vi "(nist) Post Joint Values.vi"(11 "Reply":string) -> ()   [LabVIEW 2013]
uses:
  (nist) Arm Globals.vi
panel:
  out "R":u32
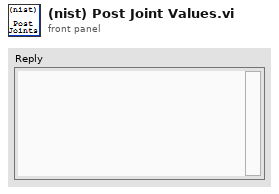
[diagram p1: front panel]
types:
  T1 = cluster{"Joint Names":string[], "Position":dbl[], "Velocity":dbl[], "Effort":dbl[]}
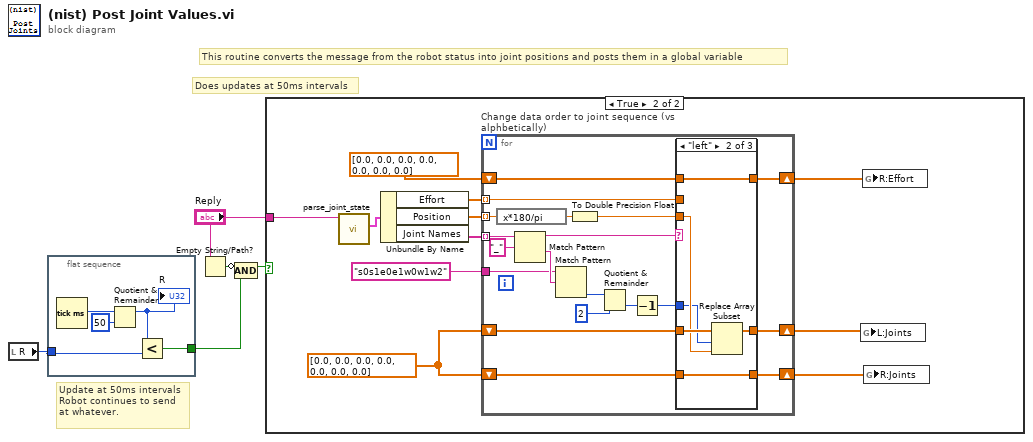
[diagram p0: block diagram]
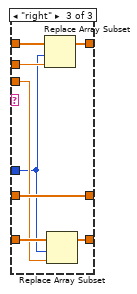
[diagram p4: hidden frame]
diagram:
  # "Update at 50ms intervals\nRobot continues to send\nat whatever."
  # "Does updates at 50ms intervals"
  # "This routine converts the message from the robot status into joint positions and posts them in a global variable"
  n1 = local read "R"() -> (w1:u32)
  n2 = flat-sequence {
    tunnel: [w7] -> w2
    tunnel: w1 -> [w6]
    frame #0 {
      n3 = Tick Count (ms)() -> (millisecond timer value=w10:u32)
      n4 = Quotient & Remainder(x=w10, y=u32 50) -> (x-y*floor(x/y)=w8:u32)  [unwired: 1 out]
      "R" <- w8
      n5 = Less?(x=w8, y=w6) -> (x < y?=w7:bool)
    }
  }
  n6 = Empty String/Path?(string/path="Reply") -> (empty?=w5:bool)
  n7 = Compound Arithmetic op=AND(invert w5, w2) -> (w3:bool)
  n8 = case shown="True" w3 {
    tunnel: "Reply" -> [_ w16]
    frame False {
    }
    frame True {
      w21 = dbl[] [0.0, 0.0, 0.0, 0.0, 0.0, 0.0, 0.0]
      n9 = call "parse_joint_state.vi"("msg in"=w16) -> ("ROS Joint States"=w19:T1)  [unwired: 3 in, 3 out]
      n10 = Unbundle By Name(w19) -> ("Effort"=w13:dbl[], "Position"=w18:dbl[], "Joint Names"=w17:string[])
      n11 = for "Change data order to joint sequence (vs alphbetically)" {
        shift-right: [w40] -> w14
        shift-left: w21 -> [w39]
        shift-right: [w37] -> w15
        shift-left: w21 -> [w38]
        tunnel: w17 -> [w33] mode=indexing
        tunnel: w18 -> [w36] mode=indexing
        tunnel: "s0s1e0e1w0w1w2" -> [w26]
        tunnel: w13 -> [w24] mode=indexing
        shift-right: [w23] -> w11
        shift-left: dbl[] [0.0, 0.0, 0.0, 0.0, 0.0, 0.0, 0.0] -> [w22]
        n12 = expression code="x*180/pi"(w36) -> (w35:dbl)
        n13 = Match Pattern(string=w33, regular expression="_") -> (before substring=w27:string, after substring=w31:string)  [unwired: 1 in, 2 out]
        n14 = Match Pattern(string=w26, regular expression=w31) -> (offset past match=w30:i32)  [unwired: 1 in, 3 out]
        n15 = To Double Precision Float(number=w35) -> (double precision float=w34:dbl)
        n16 = Quotient & Remainder(x=w30, y=2) -> (floor(x/y)=w28:i32)  [unwired: 1 out]
        n17 = Decrement(x=w28) -> (x-1=w25:i32)
        n18 = case shown="\"left\"" w27 {
          tunnel: [w43 w47 w57] -> w40
          tunnel: w39 -> [w43 w48 w57]
          tunnel: w34 -> [_ w46 w54]
          tunnel: w38 -> [w42 w49 w55]
          tunnel: [w42 w49 w56] -> w37
          tunnel: w25 -> [_ w45 w52]
          tunnel: w24 -> [_ _ w53]
          tunnel: [w41 w44 w51] -> w23
          tunnel: w22 -> [w41 w44 w50]
          frame Default {
          }
          frame "left" {
            n19 = Replace Array Subset(array=w48, new element=w46, index=w45) -> (w47:dbl[])
          }
          frame "right" {
            n20 = Replace Array Subset(array=w50, new element=w53, index=w52) -> (w51:dbl[])
            n21 = Replace Array Subset(array=w55, new element=w54, index=w52) -> (w56:dbl[])
          }
        }
      }
      n22 = global write "(nist) Arm Globals.vi" "L:Joints"(w14) -> ()
      n23 = global write "(nist) Arm Globals.vi" "R:Effort"(w11) -> ()
      n24 = global write "(nist) Arm Globals.vi" "R:Joints"(w15) -> ()
    }
  }
